vi "GT Get Capture Repeat Pos.vi"(6 "count":i16, 7 "startNum":i16, 8 "error in (no error)":errorcluster caption="错误输入（无错误）", 9 "pValue":i16[](array[numeric]), 10 "encoder":i16, 11 "cardNum":i16) -> (0 "error out":errorcluster caption="错误输出", 1 "pValue out":i16[](array[numeric]), 3 "function return":i16)   [LabVIEW 2020, in "gts.lvlib"]
doc: "GT_API GT_GetCaptureRepeatPos(short cardNum,short encoder,long *pValue,short startNum,short count);"
uses:
  gts.lvlib
  dll/32bit/multi_card/gts.dll
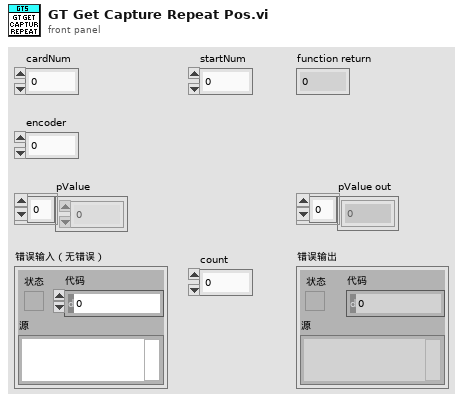
[diagram p1: front panel]
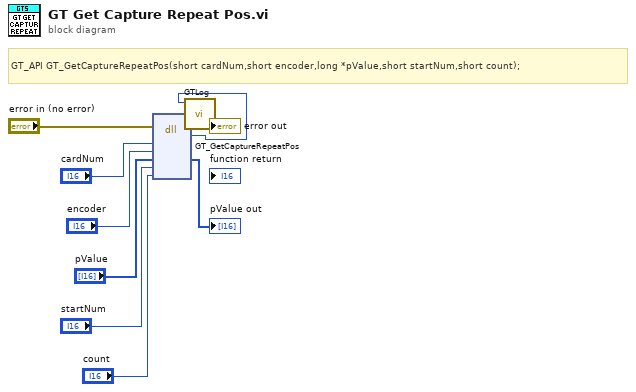
[diagram p0: block diagram]
diagram:
  # "GT_API GT_GetCaptureRepeatPos(short cardNum,short encoder,long *pValue,short startNum,short count);"
  n1 = dll-call lib="C:/1228/dll/32bit/multi_card/gts.dll" fn="GT_GetCaptureRepeatPos"(error in="error in (no error)", "cardNum"="cardNum", "encoder"="encoder", "pValue"="pValue", "startNum"="startNum", "count"="count") -> (error out=w3:errorcluster, "返回类型"=w1:i16, "pValue"=→"pValue out":i32[])  [unwired: 6 in, 1 out]
  n2 = call "GTLog.vi"("error in (no error)"=w3, "Numeric"=w1) -> ("error out"=→"error out":errorcluster)  [unwired: 9 in]
